vi "Pre Launch Init.vi"(11 "ServerUI in":refnum<class "ServerUI.lvclass">) -> (0 "error out":errorcluster, 3 "ServerUI out":refnum<class "ServerUI.lvclass">)   [LabVIEW 2018, in "ServerUI.lvlib" / "ServerUI.lvclass"]
doc: "(<B>Filename</B>: Actor Framework.lvlib:Actor.lvclass:Pre Launch Init.vi)\n\nDefines behavior that occurs after the Launch Nested Actor method is invoked but before the actor's Actor Core method begins running.\n\nBy default, this method does nothing. A descendant class may override it to define behavior."
uses:
  ServerUI.lvclass
  ServerUI.lvclass/ServerUI.ctl
  TCP_Server/TCP_Server/TCP_Server.lvclass
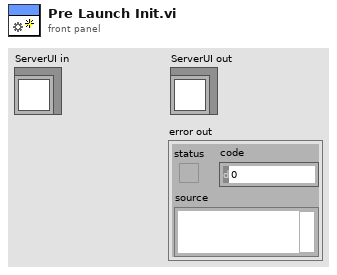
[diagram p1: front panel]
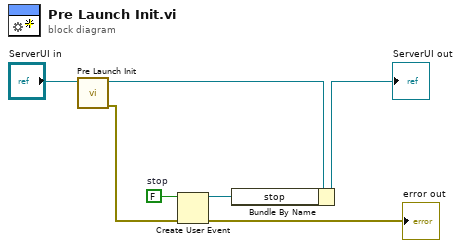
[diagram p0: block diagram]
diagram:
  w6 = FALSE  # stop
  n1 = call-parent "Pre Launch Init.vi"("Actor in"="ServerUI in") -> ("error out"=w2:errorcluster, "Actor out"=w3:refnum<class "ServerUI.lvclass">)  [unwired: 9 in]
  n2 = Create User Event(user event datatype=w6, error in=w2) -> (user event=w5:refnum<user-event>, error out=→"error out":errorcluster)
  n3 = Bundle By Name(cluster=w3, "stop"=w5) -> (→"ServerUI out":refnum<class "ServerUI.lvclass">)
